vi "Add.vi"(8 "error in (no error)":errorcluster, 9 "Value":string, 10 "Key":string, 11 "StringMap in":refnum<class "StringMap.lvclass">) -> (0 "error out":errorcluster, 3 "StringMap out":refnum<class "StringMap.lvclass">)   [LabVIEW 2013, in "LapDog.Collections.v_.Maps.lvlib" / "StringMap.lvclass"]
doc: "Add a key-value pair to the map.\n\nIf the key already exists, error 510202 is returned."
uses:
  StringMap.lvclass
  ObjectMap/ObjectMap.lvclass
  LapDog.Collections.Common/String/String.lvclass
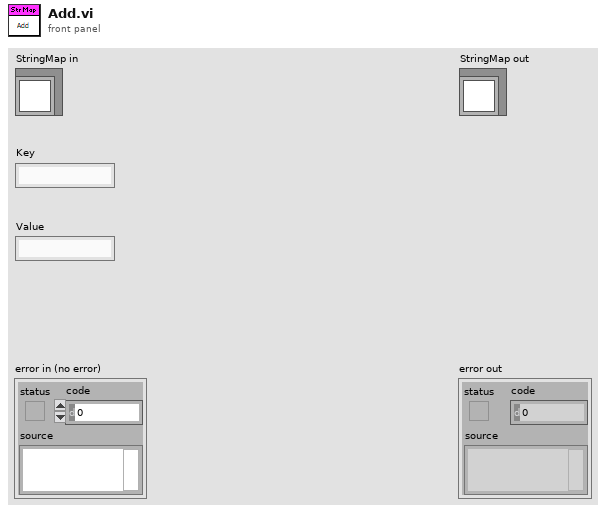
[diagram p1: front panel]
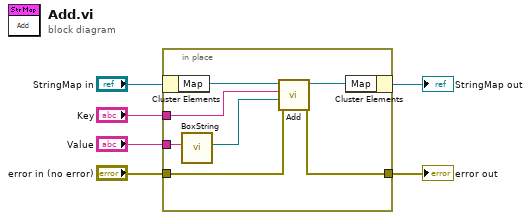
[diagram p0: block diagram]
diagram:
  n1 = in-place {
    in-place-border: "Key" -> [w12]
    in-place-border: "Value" -> [w11]
    in-place-border: "error in (no error)" -> [w9]
    in-place-border: [w8] -> w2
    n2 = in-place-cluster #1("StringMap in") -> ("Map"=w13:refnum<class "ObjectMap.lvclass">)
    n3 = call "BoxString.vi"("String"=w11) -> ("String out"=w10:refnum<class "String.lvclass">)  [unwired: 10 in]
    n4 = call-dynamic "Add.vi"("error in (no error)"=w9, "Value"=w10, "Key"=w12, "Map in"=w13) -> ("error out"=w8:errorcluster, "Map out"=w7:refnum<class "ObjectMap.lvclass">)  [unwired: 6 in]
    n5 = in-place-cluster #1("Map"=w7) -> (→"StringMap out":refnum<class "StringMap.lvclass">)
  }
  "error out" <- w2
